vi "S8300E_SetRTCTime_FromSFCS_new.vi"() -> ()   [LabVIEW 2011]
uses:
  Instance           3 34Saved   MojoMP_SetRTCTime_FromSFCS .vi
  Instance           5 34Saved   MojoMP_SetRTCTime_FromSFCS .vi
  Instance           6 34Saved   MojoMP_SetRTCTime_FromSFCS .vi
  data/MCSDLL.dll
panel:
  out "UUT Msg":string
  out "SFCS Msg":string
  out "VISA resource name out":refnum<visa-resource-name>
  out "begin time":u32
  out "toS8300E_RTC_Data":string
  out "SFCS_Time":string
  out "SFCS_DATE_STRING":string
  out "output param":string
  out "STAGE":string
  out "SFCS_IP":string
  in  "URL":string
  # "設定標準時間\nSetRTC Time from SFCS To S8300E"
  # "2014-12-15"
  # "Error Code:RTC\nError Code:UART"
  # "COM9"
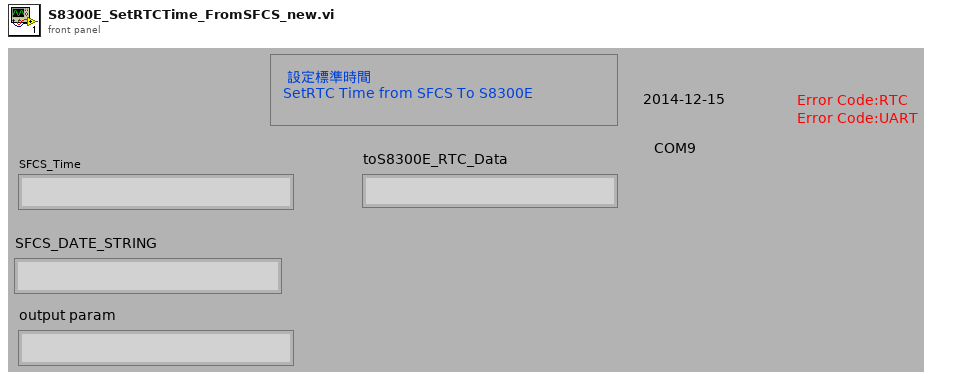
[diagram p1: front panel]
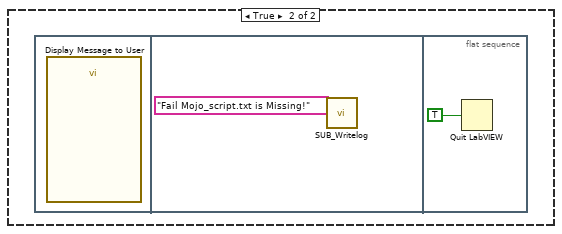
[diagram p3: hidden frame]
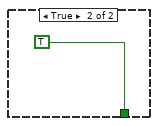
[diagram p7: hidden frame]
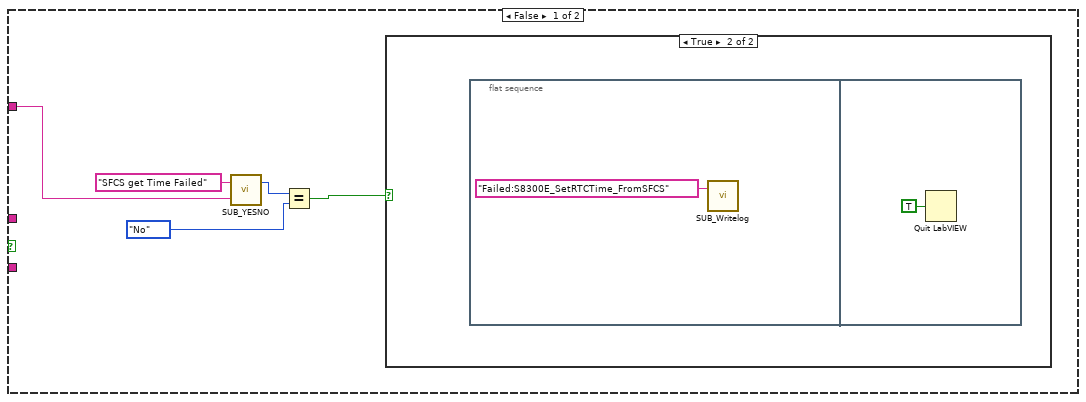
[diagram p8: hidden frame]
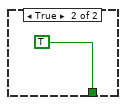
[diagram p11: hidden frame]
diagram:
  n1 = flat-sequence {
    tunnel: [w4] -> w1
    tunnel: w1 -> [w27]
    frame #0 {
      n2 = Tick Count (ms)() -> (millisecond timer value=→"begin time":u32)
    }
    frame #1 {
      n3 = call "SUB_Read_specifFile.vi"("name or relative path"="S8300E_sfcs_misc.txt" ("Script FileName")) -> ("error out"=w7:errorcluster, "text"=w4:string)  [unwired: 1 in]
      n4 = Unbundle By Name(w7) -> ("code"=w6:i32)
      n5 = Not Equal To 0?(x=w6) -> (x != 0?=w5:bool)
      n6 = case shown="False" w5 {
        tunnel: w4 -> [w8 _]
        frame False {
          n7 = flat-sequence {
            tunnel: w8 -> [w14]
            frame #0 {
              n8 = To Upper Case(1:"SFCS_IP=" ("string")) -> (0:w18:string)
              n9 = To Upper Case(1:w14) -> (0:w19:string)
              n10 = call <vilib>:"Trim Whitespace.vi"("string"=w18) -> ("trimmed string"=w16:string)  [unwired: 1 in]
              n11 = call <vilib>:"Trim Whitespace.vi"("string"=w19) -> ("trimmed string"=w15:string)  [unwired: 1 in]
              n12 = Match Pattern(string=w15, regular expression=w16) -> (after substring=w13:string)  [unwired: 1 in, 3 out]
              n13 = Match Pattern(string=w13, regular expression=";") -> (before substring=w11:string)  [unwired: 1 in, 3 out]
              "SFCS_IP" <- w11
              n14 = Equal?(x=w11, y="") -> (x = y?=w9:bool)
              n15 = case shown="True" w9 {
                frame False {
                }
                frame True {
                  n16 = flat-sequence {
                    frame #0 {
                      n17 = call "Display Message to User2"() -> ()  [unwired: 10 in, 2 out]
                    }
                    frame #1 {
                      n18 = call "SUB_Writelog.vi"("Pass/Fail"="Fail Not Found SFCS_IP=\"xx.xx.xx.xx\" in Mojo_script.txt !") -> ()  [unwired: 2 in]
                    }
                    frame #2 {
                      n19 = Quit LabVIEW(quit? (T)=TRUE) -> ()
                    }
                  }
                }
              }
            }
          }
        }
        frame True {
          n20 = flat-sequence {
            frame #0 {
              n21 = call "Display Message to User"() -> ()  [unwired: 10 in, 2 out]
            }
            frame #1 {
              n22 = call "SUB_Writelog.vi"("Pass/Fail"="Fail Mojo_script.txt is Missing!") -> ()  [unwired: 2 in]
            }
            frame #2 {
              n23 = Quit LabVIEW(quit? (T)=TRUE) -> ()
            }
          }
        }
      }
    }
    frame #2 {
      n24 = To Upper Case(1:"SFCS_STAGE=" ("string")) -> (0:w33:string)
      n25 = To Upper Case(1:w27) -> (0:w34:string)
      n26 = call <vilib>:"Trim Whitespace.vi"("string"=w33) -> ("trimmed string"=w32:string)  [unwired: 1 in]
      n27 = call <vilib>:"Trim Whitespace.vi"("string"=w34) -> ("trimmed string"=w31:string)  [unwired: 1 in]
      n28 = Match Pattern(string=w31, regular expression=w32) -> (after substring=w30:string)  [unwired: 1 in, 3 out]
      n29 = Match Pattern(string=w30, regular expression=";") -> (before substring=w26:string)  [unwired: 1 in, 3 out]
      "STAGE" <- w26
      n30 = Not Equal?(x=w26, y="") -> (x != y?=w24:bool)
      n31 = case shown="False" w24 {
        frame False {
          n32 = flat-sequence {
            frame #0 {
              n33 = call "Display Message to User4"() -> ()  [unwired: 10 in, 2 out]
            }
            frame #1 {
              n34 = call "SUB_Writelog.vi"("Pass/Fail"="Fail :Stage  not define in script file!") -> ()  [unwired: 2 in]
            }
            frame #2 {
              n35 = Quit LabVIEW(quit? (T)=TRUE) -> ()
            }
          }
        }
        frame True {
        }
      }
    }
    frame #3 {
      n36 = local read "SFCS_IP"() -> (w37:string)
      n37 = local write "URL"(w37) -> ()
    }
    frame #4 {
      n38 = call "SUB_COM1_CLOSE.vi"("VISA resource name"=refnum<visa-resource-name> "COM9") -> ()  [unwired: 3 in]
    }
    frame #5 {
      n39 = call "SUB_COM9_INIT.vi"("baud rate"=u32 115200) -> ("VISA resource name out"=w42:refnum<visa-resource-name>)  [unwired: 1 in, 1 out]
      "VISA resource name out" <- w42
      n40 = call "SUB_COM1Wrt.vi"("VISA resource name"=w42, "write buffer"="\r") -> ("duplicate VISA resource name"=w39:refnum<visa-resource-name>)  [unwired: 1 in, 1 out]
      n41 = call "SUB_ContinueCom1Read.vi"("Numeric"=1200, "duplicate VISA resource name 2"=w39) -> ()  [unwired: 1 in, 3 out]
    }
    frame #6 {
      n42 = case shown="True" TRUE {
        frame False {
        }
        frame True {
          n43 = while {
            stop <- w54 stop-if-true
            w47 = "S8300E" ("Find this String")
            w48 = "\r"
            n44 = Tick Count (ms)() -> (millisecond timer value=w51:u32)
            n45 = local read "VISA resource name out"() -> (w53:refnum<visa-resource-name>)
            n46 = Concatenate Strings(w48, w48, w48) -> (w49:string)
            n47 = call "SUB_COM1Wrt.vi"("VISA resource name"=w53, "write buffer"=w49) -> ("duplicate VISA resource name"=w52:refnum<visa-resource-name>)  [unwired: 1 in, 1 out]
            n48 = call "SUB_READ_COM1_FindString_timeout.vi"("Find this String"=w47, "Timeout Seccond"=3.0, "Begin time"=w51, "duplicate VISA resource name 2"=w52) -> ("Output String"=w46:string)  [unwired: 1 in, 2 out]
            n49 = call "SUB_FindSpecificString.vi"("Find this String"=w47, "String data"=w46) -> ("Found"=w45:bool)  [unwired: 2 in, 1 out]
            n50 = case shown="False" w45 {
              tunnel: w46 -> [w59 _]
              tunnel: [w55 TRUE] -> w54
              frame False {
                n51 = call "SUB_YESNO.vi"("Debug View"=w59, "Status"="UART無正確反應!需有S8300E字串") -> ("yes/no"=w58:enum32{"No Selection", "Yes", "No", "None"})  [unwired: 1 in]
                n52 = Equal?(x=w58, y=enum32{"No Selection", "Yes", "No", "None"}."No") -> (x = y?=w56:bool)
                n53 = case shown="True" w56 {
                  tunnel: [_ w61] -> w55
                  frame False {
                  }
                  frame True {
                    n54 = flat-sequence {
                      tunnel: [w65] -> w61
                      frame #0 {
                        n55 = call "SUB_Writelog.vi"("Pass/Fail"="Fail:S8300E_SetRTCTime_FromSFCS") -> ()  [unwired: 2 in]
                      }
                      frame #1 {
                        n56 = call "SUB_SFCS_SendResult.vi"("ErrorCode"="UART", "PASS_Fail (1/0)"=i8 0) -> ()  [unwired: 1 out]
                      }
                      frame #2 {
                        w65 = TRUE ("quit? (T)")
                        n57 = Quit LabVIEW(quit? (T)=w65) -> ()
                      }
                    }
                  }
                }
              }
              frame True {
              }
            }
          }
        }
      }
    }
    frame #7 {
      n58 = while {
        stop <- w67 stop-if-true
        w84 = ":" ("regular expression")
        w86 = "/" ("regular expression")
        w88 = " " ("regular expression")
        n59 = local read "STAGE"() -> (w92:string)
        n60 = To Upper Case(1:"NG" ("string")) -> (0:w99:string)
        n61 = To Upper Case(1:"Fail" ("string")) -> (0:w76:string)
        n62 = call <vilib>:"Trim Whitespace.vi"("string"=w99) -> ("trimmed string"=w96:string)  [unwired: 1 in]
        n63 = call <vilib>:"Trim Whitespace.vi"("string"=w76) -> ("trimmed string"=w73:string)  [unwired: 1 in]
        n64 = dll-call lib="D:/S8300E_Project/data/MCSDLL.dll" fn="SFCS_GetCurrentDBSysdate"("URL"="URL", "Stage"=w92, "TimeFormat"="YYYY/MM/DD HH24:MI:SS") -> (w68:string)  [unwired: 6 in, 2 out]
        "output param" <- w68
        "SFCS Msg" <- w68
        n65 = To Upper Case(1:w68) -> (0:w100:string)
        n66 = To Upper Case(1:w68) -> (0:w77:string)
        n67 = call <vilib>:"Trim Whitespace.vi"("string"=w100) -> ("trimmed string"=w95:string)  [unwired: 1 in]
        n68 = call <vilib>:"Trim Whitespace.vi"("string"=w77) -> ("trimmed string"=w72:string)  [unwired: 1 in]
        n69 = Match Pattern(string=w95, regular expression=w96) -> (match substring=w97:string)  [unwired: 1 in, 3 out]
        n70 = Match Pattern(string=w72, regular expression=w73) -> (match substring=w74:string)  [unwired: 1 in, 3 out]
        n71 = Not Equal?(x=w97, y=w96) -> (x != y?=w71:bool)
        n72 = Not Equal?(x=w74, y=w73) -> (x != y?=w70:bool)
        n73 = Match Pattern(string=w68, regular expression=w84) -> (match substring=w85:string)  [unwired: 1 in, 3 out]
        n74 = Match Pattern(string=w68, regular expression=w86) -> (match substring=w87:string)  [unwired: 1 in, 3 out]
        n75 = And(x=w71, y=w70) -> (x .and. y?=w69:bool)
        n76 = Equal?(x=w87, y=w86) -> (x = y?=w81:bool)
        n77 = Equal?(x=w85, y=w84) -> (x = y?=w83:bool)
        n78 = Match Pattern(string=w68, regular expression=w88) -> (before substring=w91:string, match substring=w89:string, after substring=w90:string)  [unwired: 1 in, 1 out]
        n79 = And(x=w83, y=w69) -> (x .and. y?=w79:bool)
        n80 = Equal?(x=w89, y=w88) -> (x = y?=w82:bool)
        n81 = And(x=w82, y=w81) -> (x .and. y?=w80:bool)
        n82 = And(x=w80, y=w79) -> (x .and. y?=w78:bool)
        n83 = case shown="True" w78 {
          tunnel: w91 -> [_ w111]
          tunnel: w90 -> [_ w110]
          tunnel: w68 -> [w101 _]
          tunnel: [_ w109] -> w67
          frame False {
            n84 = call "SUB_YESNO.vi"("Debug View"=w101, "Status"="SFCS get Time Failed") -> ("yes/no"=w104:enum32{"No Selection", "Yes", "No", "None"})  [unwired: 1 in]
            n85 = Equal?(x=w104, y=enum32{"No Selection", "Yes", "No", "None"}."No") -> (x = y?=w102:bool)
            n86 = case shown="True" w102 {
              frame False {
              }
              frame True {
                n87 = flat-sequence {
                  frame #0 {
                    n88 = call "SUB_Writelog.vi"("Pass/Fail"="Failed:S8300E_SetRTCTime_FromSFCS") -> ()  [unwired: 2 in]
                  }
                  frame #1 {
                    n89 = Quit LabVIEW(quit? (T)=TRUE) -> ()
                  }
                }
              }
            }
          }
          frame True {
            n90 = flat-sequence {
              tunnel: w111 -> [w127]
              tunnel: w110 -> [w126]
              tunnel: [w112] -> w108
              tunnel: [w136] -> w109
              tunnel: w108 -> [w134]
              frame #0 {
                n91 = call <vilib>:"Trim Whitespace.vi"("string"=w127) -> ("trimmed string"=w118:string)  [unwired: 1 in]
                "SFCS_DATE_STRING" <- w118
                n92 = call <vilib>:"Trim Whitespace.vi"("string"=w126) -> ("trimmed string"=w125:string)  [unwired: 1 in]
                "SFCS_Time" <- w125
                n93 = call "SUB_OUT_THIS_token.vi"("Remove token symbl1 3"="", "Remove token symbl1 2"=":" ("Remove token symbl1"), "Remove token symbl1"="/", "input string"=w125) -> ("result string"=w116:string)  [unwired: 1 in]
                n94 = call "SUB_OUT_THIS_token.vi"("Remove token symbl1 3"="", "Remove token symbl1 2"=":" ("Remove token symbl1"), "Remove token symbl1"="/", "input string"=w118) -> ("result string"=w117:string)  [unwired: 1 in]
                n95 = Concatenate Strings(w117, w116) -> (w113:string)
                "toS8300E_RTC_Data" <- w113
                n96 = Concatenate Strings("./rtc.sh -w  ", w113, "\r") -> (w112:string)
              }
              frame #1 {
                n97 = local read "VISA resource name out"() -> (w135:refnum<visa-resource-name>)
                n98 = Tick Count (ms)() -> (millisecond timer value=w130:u32)
                n99 = call "SUB_COM1Wrt.vi"("VISA resource name"=w135, "write buffer"=w134) -> ("duplicate VISA resource name"=w133:refnum<visa-resource-name>)  [unwired: 1 in, 1 out]
                n100 = call "SUB_COM_NoErrRead_TimeOut.vi"("Timeout Seccond"=5.0, "Begin time"=w130, "Find this String"="PASSED=", "VISA resource name"=w133) -> ("concatenated string"=→"UUT Msg":string, "Found"=w132:bool)  [unwired: 4 in]
                n101 = case shown="False" w132 {
                  tunnel: [_ TRUE] -> w136
                  frame False {
                    n102 = local read "UUT Msg"() -> (w140:string)
                    n103 = call "SUB_YESNO.vi"("Debug View"=w140, "Status"="設定RTC失敗!") -> ("yes/no"=w139:enum32{"No Selection", "Yes", "No", "None"})  [unwired: 1 in]
                    n104 = Equal?(x=w139, y=enum32{"No Selection", "Yes", "No", "None"}."No") -> (x = y?=w137:bool)
                    n105 = case shown="True" w137 {
                      frame False {
                      }
                      frame True {
                        n106 = flat-sequence {
                          frame #0 {
                            n107 = call "SUB_SFCS_SendResult.vi"("ErrorCode"="RTC", "PASS_Fail (1/0)"=i8 0) -> ()  [unwired: 1 out]
                          }
                          frame #1 {
                            n108 = call "SUB_Writelog.vi"("Pass/Fail"="Failed:S8300E_SetRTCTime_FromSFCS") -> ()  [unwired: 2 in]
                          }
                          frame #2 {
                            n109 = Quit LabVIEW(quit? (T)=TRUE) -> ()
                          }
                        }
                      }
                    }
                  }
                  frame True {
                  }
                }
              }
            }
          }
        }
      }
    }
    frame #8 {
      n110 = call "SUB_COM1_CLOSE.vi"("VISA resource name"=refnum<visa-resource-name> "COM9") -> ()  [unwired: 3 in]
    }
    frame #9 {
      w150 = "\r"
      n111 = local read "SFCS Msg"() -> (w153:string)
      n112 = local read "UUT Msg"() -> (w151:string)
      n113 = Tick Count (ms)() -> (millisecond timer value=w157:u32)
      n114 = local read "begin time"() -> (w158:u32)
      n115 = call "SUB_CAL_TESTTIME.vi"("Test Item name"="S8300E_SetRTCTime_FromSFCS", "Stop tick time"=w157, "Start tick time"=w158) -> ("Test Time output"=w149:string)  [unwired: 2 in]
      n116 = Concatenate Strings("Pass :S8300E_SetRTCTime_FromSFCS" ("Pass/Fail"), w150, "SFCS Message:", w153, w150, "UUT Message:", w151, w150, w149) -> (w148:string)
      n117 = call "SUB_Writelog.vi"("Pass/Fail"=w148) -> ()  [unwired: 2 in]
    }
    frame #10 {
      n118 = Request Deallocation(TRUE ("flag")) -> ()
    }
    frame #11 {
      n119 = Quit LabVIEW(quit? (T)=TRUE) -> ()
    }
  }
